vi "From RP I-V to Lockin.vi"(7 "Lockin Configuration in":T3={"Post-trigger delay"=0.01, "Post-trigger duration"=0.1, "Rate"=1000000.0, "Ranges"=[10.0], "Re-name channels"=[], "Active channels"="0:1", "External\nclock"=FALSE, "Frequencies"=[], "Monitor time\nconstant"=1.0, "Output \namplitudes"=[], "Input\nchannles"=[], "Sync"=FALSE, "Lock-in input channel phases"=[]} {"Output \namplitudes" format="%#_6pV"; "Monitor time\nconstant" format="%#_6ps"; "Frequencies" format="%#_6pHz"; "Rate" format="%#_8pHz"; "Post-trigger duration" format="%#_6ps"; "Post-trigger delay" format="%#_6ps"; "Ranges" format="%#_6pV"}, 10 "Rate":dbl=125000000.0 format="%#_6pHz", 11 "Configuration":T1={"I-V parameters"={"Start magnitude"=0.0, "Magnitude increment"=0.0, "End magnitude"=0.0, "Ramp length"=0, "Top  length"=0, "Threshold "=0.0, "Processing delay"=0, "Output gain "=0.0, "Interpolation"=0, "Stop after"=1, "Detector window"=480}, "Ranges"=[], "Post-trigger delay"=0.01, "Post-trigger duration"=0.1, "Output delay"=0.1} {"Output delay" format="%#_6ps"; "Post-trigger duration" format="%#_6ps"; "Post-trigger delay" format="%#_6ps"; "Ranges" format="%#_6pV"; "I-V parameters"."Detector window" format="%dpts"; "I-V parameters"."Stop after" format="%d sweep(s)"; "I-V parameters"."Output gain" format="%#_6pA/V"; "I-V parameters"."Processing delay" format="%dpts"; "I-V parameters"."Threshold" format="%#_6pV"; "I-V parameters"."Top  length" format="%dpts"; "I-V parameters"."Ramp length" format="%dpts"; "I-V parameters"."End magnitude" format="%#_6pA"; "I-V parameters"."Magnitude increment" format="%#_6pA"; "I-V parameters"."Start magnitude" format="%#_6pA"}) -> (3 "Lockin Configuration out":T3={"Post-trigger delay"=0.01, "Post-trigger duration"=0.1, "Rate"=1000000.0, "Ranges"=[10.0], "Re-name channels"=[], "Active channels"="0:1", "External\nclock"=FALSE, "Frequencies"=[], "Monitor time\nconstant"=1.0, "Output \namplitudes"=[], "Input\nchannles"=[], "Sync"=FALSE, "Lock-in input channel phases"=[]} {"Output \namplitudes" format="%#_6pV"; "Monitor time\nconstant" format="%#_6ps"; "Frequencies" format="%#_6pHz"; "Rate" format="%#_8pHz"; "Post-trigger duration" format="%#_6ps"; "Post-trigger delay" format="%#_6ps"; "Ranges" format="%#_6pV"})   [LabVIEW 2021]
uses:
  Instruments/Pulse Driver/Lockin Digitizer Driver/Lockin Digitizer Configuration.ctl
  Waform generation/I-V parameters.ctl
  RP I-V Configuration.ctl
panel:
  # "Waveform parameters"
  # "Detector parameters"
  # "Pulse config"
  # "Lock-in config"
  # "#0\n\n#1"
  # "Monitor config"
  # "Pulse config"
  # "Lock-in config"
  # "#0\n\n#1"
  # "Monitor config"
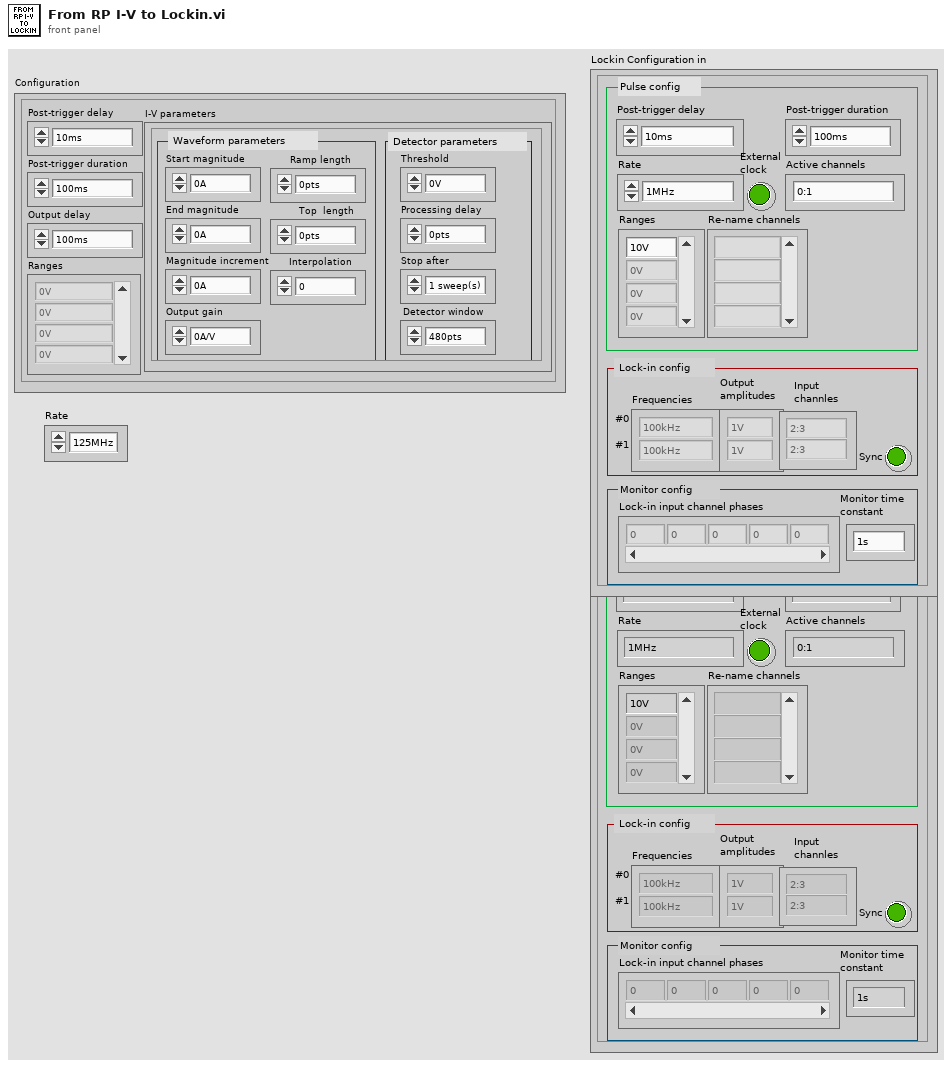
[diagram p1: front panel]
types:
  T1 = typedef "RP I-V Configuration.ctl" = cluster{"I-V parameters":T2, "Ranges":dbl[], "Post-trigger delay":dbl, "Post-trigger duration":dbl, "Output delay":dbl}
  T2 = typedef "I-V parameters.ctl" = cluster{"Start magnitude":dbl, "Magnitude increment":dbl, "End magnitude":dbl, "Ramp length":i32, "Top  length":i32, "Threshold ":dbl, "Processing delay":u16, "Output gain ":dbl, "Interpolation":i32, "Stop after":u16, "Detector window":i32}
  T3 = typedef "Lockin Digitizer Configuration.ctl" = cluster{"Post-trigger delay":dbl, "Post-trigger duration":dbl, "Rate":dbl, "Ranges":dbl[], "Re-name channels":string[], "Active channels":string, "External\nclock":bool, "Frequencies":dbl[], "Monitor time\nconstant":dbl, "Output \namplitudes":dbl[], "Input\nchannles":string[], "Sync":bool, "Lock-in input channel phases":dbl[]}
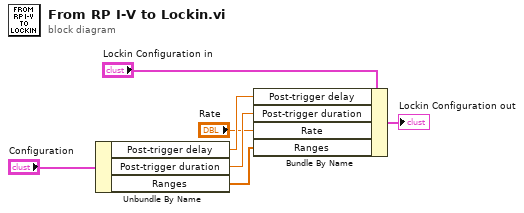
[diagram p0: block diagram]
diagram:
  n1 = Unbundle By Name("Configuration") -> ("Post-trigger delay"=w4:dbl, "Post-trigger duration"=w3:dbl, "Ranges"=w1:dbl[])
  n2 = Bundle By Name(cluster="Lockin Configuration in", "Post-trigger delay"=w4, "Post-trigger duration"=w3, "Rate"="Rate", "Ranges"=w1) -> (→"Lockin Configuration out":T3)
